vi "Dual Chronometer-RT Host.vi"() -> ()   [LabVIEW 2013]
doc: "Dual Chronometer- Works with FPGA code to sample gated transitions on digital inputs UUT1-6, REF 1-10 and writes values of interest to MODBUS registers. See documentation for list of registers that are written by this software."
uses:
  RT_host_vars.ctl
  <vilib>/Platform/TimedLoop/XDataNode/timing_clust.ctl
  <vilib>/Platform/TimedLoop/XDataNode/nitl_modes.ctl
  <vilib>/Platform/TimedLoop/XDataNode/wakeup.ctl
  <vilib>/FPGAPlugInAG/cRIO-9075/niLvFpga_Open_cRIO-9075.vi
  <vilib>/Utility/error.llb/Error Cluster From Error Code.vi
  <vilib>/rvi/errors/niLvFpgaAdjustHostInterfaceError.vi
  <vilib>/FPGAPlugInAG/cRIO-9075/niLvFpga_Close_cRIO-9075.vi
  <vilib>/Platform/TimedLoop/XDataNode/XDataNode.xnode
  <vilib>/rvi/interface/nirviOpenFPGA/nirviOpenFPGA.xnode
  FPGA Bitfiles/Calibrator_FPGATarget_FPGA-Samplecurre_Fyu26Q6DgO4.lvbitx
  FPGA-Sample_currents_read_fractional_pulses.vi
  <vilib>/rvi/interface/nirviReadWriteControl/nirviReadWriteControl.xnode
  <vilib>/rvi/interface/nirviCloseFPGA/nirviCloseFPGA.xnode
  <vilib>/Platform/TimedLoop/XDataNode/XDNodeRunTimeDep.lvlib
  NiFpgaLv.dll
panel:
  out "Sampling in progress":bool
  out "RT host variables":T1
  out "Sample period(s)":dbl
  out "Begin pulse sampling":bool
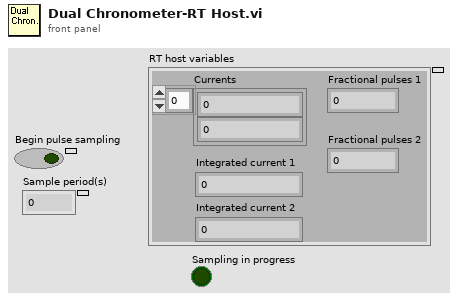
[diagram p1: front panel]
types:
  T1 = typedef "RT_host_vars.ctl" = cluster{"Fractional pulses 1":dbl, "Currents":dbl[], "Fractional pulses 2":dbl, "Integrated current 1":dbl, "Integrated current 2":dbl}
  T2 = typedef "XDNodeRunTimeDep.lvlib/timing_clust.ctl" = cluster{"Expected End [f-1]":u64, "Actual End [f-1]":u64, "Finished Late? [f-1]":bool, "Expected End [i-1]":u64, "Actual End [i-1]":u64, "Finished Late? [i-1]":bool, "Expected Start [i]":u64, "Actual Start [i]":u64, "Expected Start [f]":u64, "Actual Start [f]":u64, "Source Name":string, "Structure Name":string, "Period":i64, "Deadline":i64, "Offset":i64, "Start":i64, "Priority":i32, "Timeout":i32, "Mode":T3, "Wakeup Reason":T4, "Error":errorcluster, "Source Type":string, "Secondary Source Type":string, "Global End Time":u64, "Global Start Time":u64, "Frame Duration":u64, "Iteration Duration":u64, "Assigned CPU":i32, "I/O Scan Engine Mode":u32}
  T3 = typedef "XDNodeRunTimeDep.lvlib/nitl_modes.ctl" = enum32{"No Change", "Process missed periods, maintain original phase", "Discard missed periods, maintain original phase", "Process missed periods, ignore original phase", "Discard missed periods, ignore original phase"}
  T4 = typedef "XDNodeRunTimeDep.lvlib/wakeup.ctl" = enum32{"Normal", "Aborted", "Asynchronous wakeup", "Timing source error", "Timed loop error", "Timeout"}
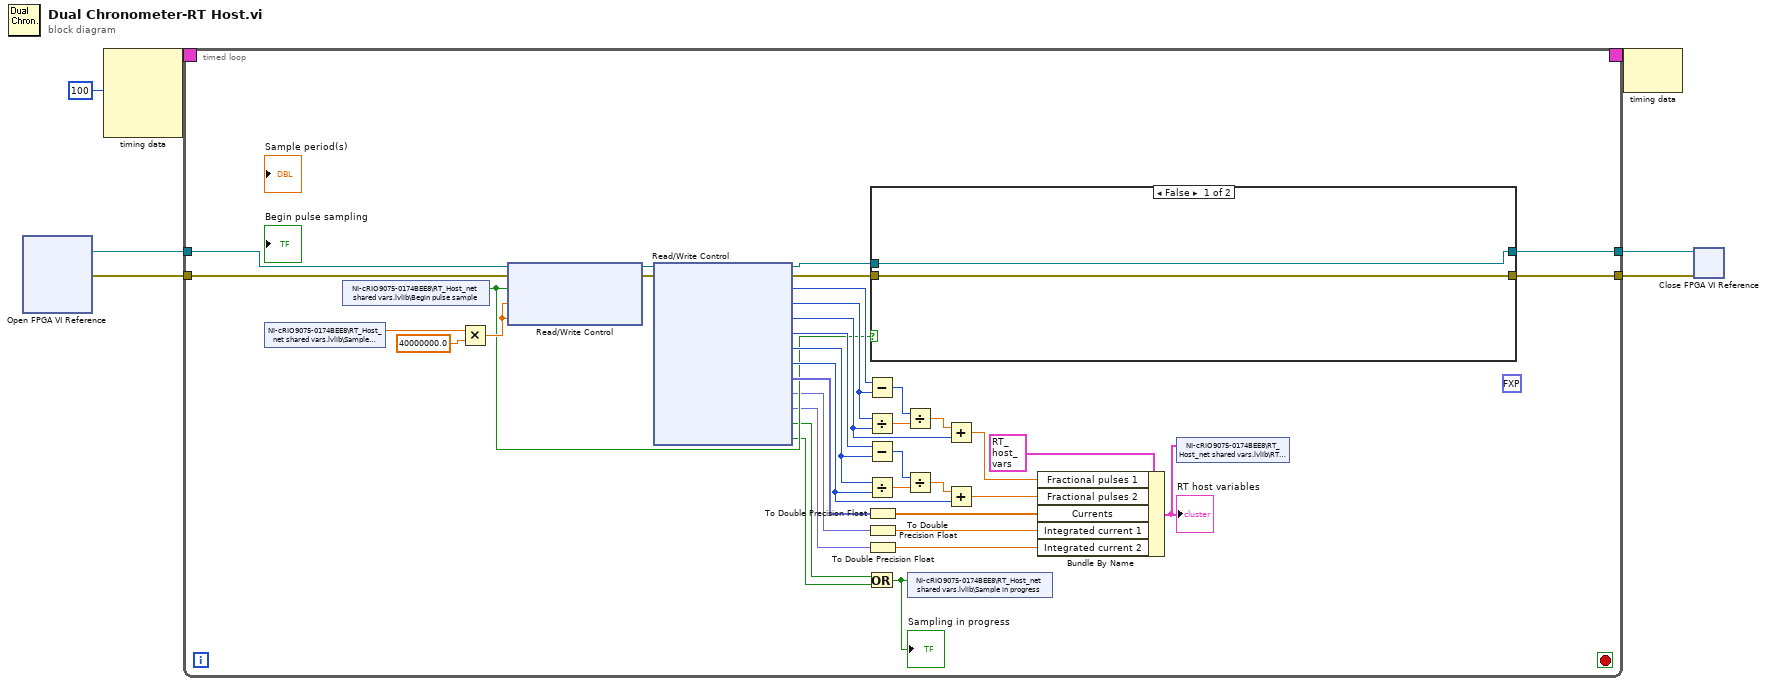
[diagram p0: block diagram]
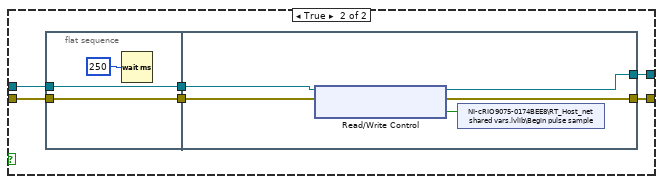
[diagram p2: hidden frame]
diagram:
  n1 = xnode "Open FPGA VI Reference"() -> ("FPGA VI Reference Out"=w3:refnum<k20>, "error out"=w2:errorcluster)  [unwired: 2 in]
  n2 = node-c288(i64 100 ("Period")) -> (w5:T2)  [unwired: 3 out]
  n3 = timed-loop {
    tunnel: w3 -> [w22]
    tunnel: w2 -> [w20]
    tunnel: [w24] -> w7
    tunnel: [w23] -> w6
    timing: w5 -> [_]
    timing-out: [_] -> w4
    stop <- _ stop-if-true
    (unwired) fxp<+/-,32,16> 0.0 ("fixed-point type")
    n4 = shared-variable "NI-cRIO9075-0174BEE8\\RT_Host_net shared vars.lvlib\\Sample period"() -> (w17:dbl)  [unwired: 1 in, 1 out]
    n5 = shared-variable "NI-cRIO9075-0174BEE8\\RT_Host_net shared vars.lvlib\\Begin pulse sample"() -> (w14:bool)  [unwired: 1 in, 1 out]
    n6 = Multiply(x=w17, y=40000000.0) -> (x*y=w18:dbl)
    n7 = xnode "Read/Write Control"("FPGA VI Reference In"=w22, "error in"=w20, "Begin pulse sampling"=w14, "Sample period Input 0"=w18, "Sample period Input 1"=w18) -> ("FPGA VI Reference Out"=w21:refnum<k20>, "error out"=w19:errorcluster)
    n8 = xnode "Read/Write Control"("FPGA VI Reference In"=w21, "error in"=w19) -> ("FPGA VI Reference Out"=w26:refnum<k20>, "error out"=w25:errorcluster, "Gate time 1"=w28:u64, "whole pulse time 1"=w44:u64, "Whole pulses 1"=w40:u64, "Gate time 2"=w27:u64, "whole pulse time 2"=w35:u64, "Whole pulses 2"=w34:u64, "Currents"=w30:fxp<+/-,24,-4>[], "mA*seconds (input 1)"=w11:fxp<+/-,64,28>, "mA*seconds (input 2)"=w10:fxp<+/-,64,28>, "Sampling in progress 1"=w13:bool, "Sampling in progress 2"=w12:bool)
    n9 = Subtract(x=w28, y=w44) -> (x-y=w43:u64)
    n10 = Divide(x=w44, y=w40) -> (x/y=w42:dbl)
    n11 = Subtract(x=w27, y=w35) -> (x-y=w36:u64)
    n12 = Divide(x=w35, y=w34) -> (x/y=w37:dbl)
    n13 = Or(x=w13, y=w12) -> (x .or. y?=w15:bool)
    "Sampling in progress" <- w15
    n14 = To Double Precision Float(number=w30) -> (double precision float=w29:dbl[])
    n15 = To Double Precision Float(number=w11) -> (double precision float=w9:dbl)
    n16 = To Double Precision Float(number=w10) -> (double precision float=w8:dbl)
    n17 = case shown="False" w14 {
      tunnel: w26 -> [w46 w52]
      tunnel: w25 -> [w45 w51]
      tunnel: [w46 w50] -> w24
      tunnel: [w45 w49] -> w23
      frame False {
      }
      frame True {
        n18 = flat-sequence {
          tunnel: w51 -> [w54]
          tunnel: w52 -> [w55]
          tunnel: [w55] -> w48
          tunnel: [w54] -> w47
          tunnel: [w58] -> w50
          tunnel: [w57] -> w49
          tunnel: w48 -> [w60]
          tunnel: w47 -> [w59]
          frame #0 {
            n19 = Wait (ms)(milliseconds to wait=u32 250) -> ()  [unwired: 1 out]
          }
          frame #1 {
            n20 = xnode "Read/Write Control"("FPGA VI Reference In"=w60, "error in"=w59) -> ("FPGA VI Reference Out"=w58:refnum<k20>, "error out"=w57:errorcluster, "Begin pulse sampling"=w56:bool)
            n21 = shared-variable "NI-cRIO9075-0174BEE8\\RT_Host_net shared vars.lvlib\\Begin pulse sample"(w56) -> ()  [unwired: 1 in, 1 out]
          }
        }
      }
    }
    n22 = Divide(x=w43, y=w42) -> (x/y=w41:dbl)
    n23 = Divide(x=w36, y=w37) -> (x/y=w38:dbl)
    n24 = shared-variable "NI-cRIO9075-0174BEE8\\RT_Host_net shared vars.lvlib\\Sample in progress"(w15) -> ()  [unwired: 1 in, 1 out]
    n25 = Add(x=w41, y=w40) -> (x+y=w33:dbl)
    n26 = Add(x=w38, y=w34) -> (x+y=w31:dbl)
    n27 = Bundle By Name(cluster=T1 {"Fractional pulses 1"=0.0, "Currents"=[0.0, 0.0, 0.0, 0.0, 0.0], "Fractional pulses 2"=0.0, "Integrated current 1"=0.0, "Integrated current 2"=0.0} ("input cluster"), "Fractional pulses 1"=w33, "Fractional pulses 2"=w31, "Currents"=w29, "Integrated current 1"=w9, "Integrated current 2"=w8) -> (w16:T1)
    "RT host variables" <- w16
    n28 = shared-variable "NI-cRIO9075-0174BEE8\\RT_Host_net shared vars.lvlib\\RT_host_vars"(w16) -> ()  [unwired: 1 in, 1 out]
  }
  n29 = node-c288(w4) -> ()  [unwired: 1 out]
  n30 = xnode "Close FPGA VI Reference"("FPGA VI Reference In"=w7, "error in"=w6) -> ()  [unwired: 1 out]
